vi "Log.vi"(8 "error in (no error)":errorcluster, 9 "Timestamp data points":bool, 10 "tdms file":refnum<k34>, 11 "File Path Result in":refnum<class "File Path Result.lvclass">) -> (0 "error out":errorcluster, 2 "tdms file out":refnum<k34>, 3 "File Path Result out":refnum<class "File Path Result.lvclass">)   [LabVIEW 2019, in "File Path Result.lvclass"]
uses:
  File Path Result.lvclass
  C:/GitHub/NHMFL_Core/Libraries/Instruments/Results/Acquired Result/Acquired Result.lvclass
  Acquired Result/Acquired Result.lvclass/Acquired Result.ctl
  Acquired Result/Read Group.vi
  Acquired Result/Acquired Result.lvclass
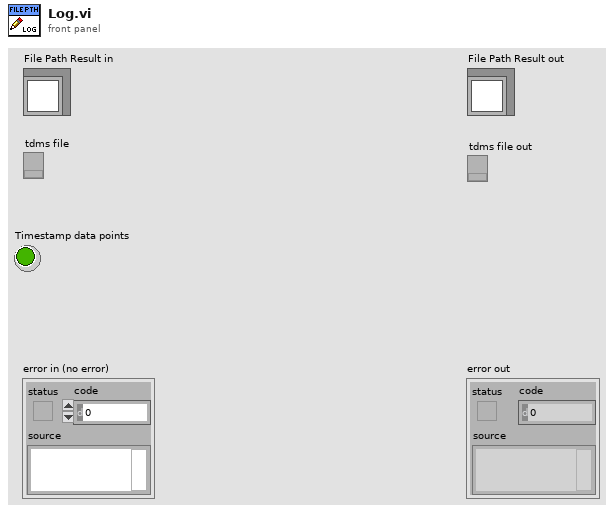
[diagram p1: front panel]
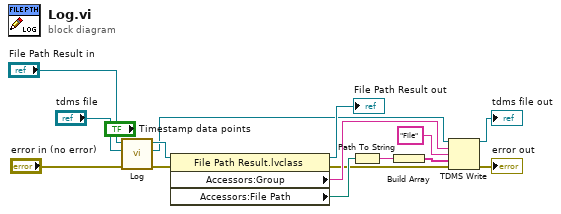
[diagram p0: block diagram]
diagram:
  n1 = call-parent "Log.vi"("error in (no error)"="error in (no error)", "tdms file"="tdms file", "Acquired Result in"="File Path Result in") -> ("error out"=w14:errorcluster, "tdms file out"=w8:refnum<k34>, "Acquired Result out"=w11:refnum<class "File Path Result.lvclass">)  [unwired: 6 in]
  n2 = property class="File Path Result.lvclass"(reference=w11, error in=w14) -> (reference out=→"File Path Result out":refnum<class "File Path Result.lvclass">, error out=w2:errorcluster, "Accessors:Group"=w6:string, "Accessors:File Path"=w9:path)
  n3 = Path To String(path=w9) -> (string=w5:string)
  n4 = Build Array(w5) -> (w4:string[])
  n5 = TDMS Write(0:w8, 5:w6, 7:"File", 9:w4, 11:w2) -> (4:→"tdms file out":refnum<k34>, 15:→"error out":errorcluster)  [unwired: 1 in, 2 out]
